vi "Int bottom stacking.vi"() -> (10 "Done":bool)   [LabVIEW 2014]
uses:
  Int Bottom Stacking.ctl
  Bottom Stacking.ctl
panel:
  in  "Int Bottom Stacking":T1
  out "Timer":dbl
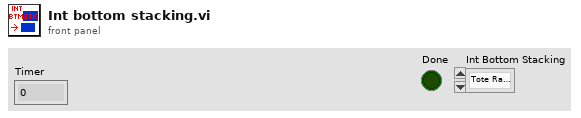
[diagram p1: front panel]
types:
  T1 = typedef "Int Bottom Stacking.ctl" = enum16{"Tote Raising", "Obtaining", "Un-Obtaining", "Tote Lowering", "Tote Release"}
  T2 = typedef "Bottom Stacking.ctl" = enum16{"Tote Raising", "Ejecting", "Un-Ejecting", "Tote Lowering", "Tote Release", "Backing Up"}
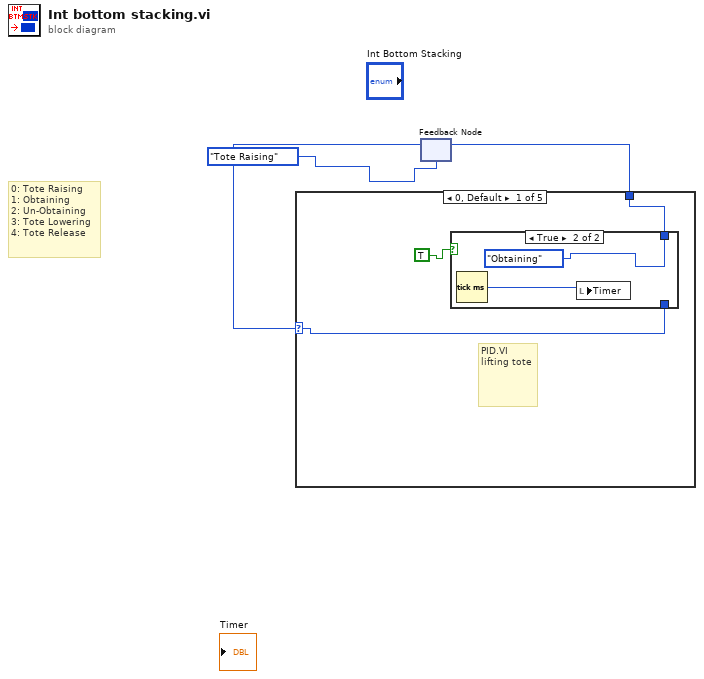
[diagram p0: block diagram]
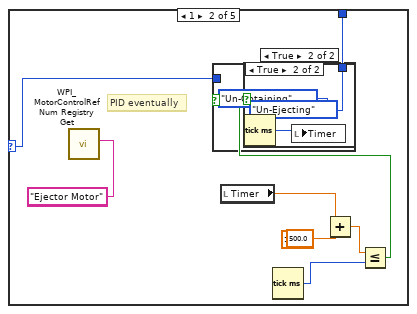
[diagram p3: hidden frame]
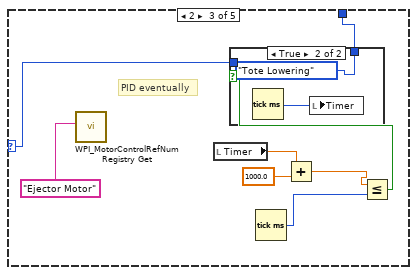
[diagram p6: hidden frame]
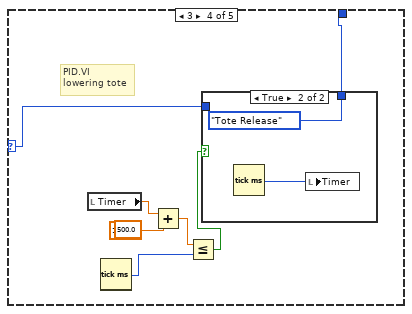
[diagram p8: hidden frame]
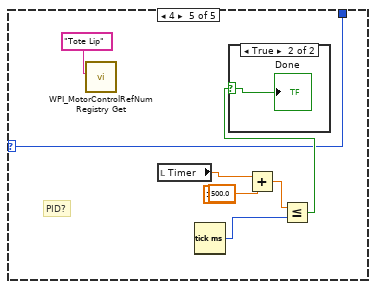
[diagram p10: hidden frame]
diagram:
  # "0: Tote Raising\n1: Obtaining\n2: Un-Obtaining\n3: Tote Lowering\n4: Tote Release"
  n1 = feedback #1(Int_Bottom_Stacking."Tote Raising" ("Int Bottom Stacking")) -> (w3:u16)
  n2 = case shown="0, Default" w3 {
    selector: w3 -> [w5 w10 w27 w37 w47]
    tunnel: [w6 w11 w29 w43 w47] -> w2
    frame 0, Default {
      # "PID.VI\nlifting tote"
      n3 = case shown="True" TRUE {
        tunnel: [w7 Int_Bottom_Stacking."Obtaining" ("Int Bottom Stacking")] -> w6
        tunnel: w5 -> [w7 _]
        frame False {
        }
        frame True {
          n4 = Tick Count (ms)() -> (millisecond timer value=w9:u32)
          n5 = local write "Timer"(w9) -> ()
        }
      }
    }
    frame 1 {
      (unwired) "Ejector Motor" ("refnum name")
      # "PID eventually"
      # "PID eventually"
      n6 = call <vilib>:"WPI_MotorControlRefNum Registry Get.vi"("refnum name"="Ejector Motor") -> ()  [unwired: 9 in, 2 out]
      n7 = local read "Timer"() -> (w21:dbl)
      n8 = local read "Timer"() -> (w12:dbl)
      n9 = Tick Count (ms)() -> (millisecond timer value=w18:u32)
      n10 = Tick Count (ms)() -> (millisecond timer value=w15:u32)
      n11 = Add(x=w21, y=500.0) -> (x+y=w19:dbl)
      n12 = Add(x=w12, y=1000.0) -> (x+y=w14:dbl)
      n13 = Less Or Equal?(x=w19, y=w18) -> (x <= y?=w17:bool)
      n14 = case shown="True" w17 {
        frame False {
        }
        frame True {
          (unwired) Bottom_Stacking."Un-Ejecting" ("Bottom Stacking")
        }
      }
      n15 = Less Or Equal?(x=w14, y=w15) -> (x <= y?=w16:bool)
      n16 = case shown="True" w16 {
        tunnel: [w23 Int_Bottom_Stacking."Un-Obtaining" ("Int Bottom Stacking")] -> w11
        tunnel: w10 -> [w23 _]
        frame False {
        }
        frame True {
          n17 = Tick Count (ms)() -> (millisecond timer value=w25:u32)
          n18 = local write "Timer"(w25) -> ()
        }
      }
    }
    frame 2 {
      # "PID eventually"
      n19 = call <vilib>:"WPI_MotorControlRefNum Registry Get.vi"("refnum name"="Ejector Motor") -> ()  [unwired: 9 in, 2 out]
      n20 = local read "Timer"() -> (w33:dbl)
      n21 = Tick Count (ms)() -> (millisecond timer value=w30:u32)
      n22 = Add(x=w33, y=1000.0) -> (x+y=w31:dbl)
      n23 = Less Or Equal?(x=w31, y=w30) -> (x <= y?=w28:bool)
      n24 = case shown="True" w28 {
        tunnel: [w34 Int_Bottom_Stacking."Tote Lowering" ("Int Bottom Stacking")] -> w29
        tunnel: w27 -> [w34 _]
        frame False {
        }
        frame True {
          n25 = Tick Count (ms)() -> (millisecond timer value=w36:u32)
          n26 = local write "Timer"(w36) -> ()
        }
      }
    }
    frame 3 {
      (unwired) 500.0 ("y")
      # "PID.VI\nlowering tote"
      n27 = local read "Timer"() -> (w39:dbl)
      n28 = Tick Count (ms)() -> ()  [unwired: 1 out]
      n29 = Tick Count (ms)() -> (millisecond timer value=w40:u32)
      n30 = Add(x=w39, y=1000.0) -> (x+y=w41:dbl)
      n31 = Less Or Equal?(x=w41, y=w40) -> (x <= y?=w38:bool)
      n32 = case shown="True" w38 {
        tunnel: [w44 Int_Bottom_Stacking."Tote Release" ("Int Bottom Stacking")] -> w43
        tunnel: w37 -> [w44 _]
        frame False {
        }
        frame True {
          n33 = Tick Count (ms)() -> (millisecond timer value=w46:u32)
          n34 = local write "Timer"(w46) -> ()
        }
      }
    }
    frame 4 {
      (unwired) 1000.0 ("y")
      # "PID?"
      n35 = call <vilib>:"WPI_MotorControlRefNum Registry Get.vi"("refnum name"="Tote Lip") -> ()  [unwired: 9 in, 2 out]
      n36 = local read "Timer"() -> (w49:dbl)
      n37 = Tick Count (ms)() -> (millisecond timer value=w52:u32)
      n38 = Tick Count (ms)() -> ()  [unwired: 1 out]
      n39 = Add(x=w49, y=500.0) -> (x+y=w51:dbl)
      n40 = Less Or Equal?(x=w51, y=w52) -> (x <= y?=w48:bool)
      n41 = case shown="True" w48 {
        selector: w48 -> [_ w54]
        frame False {
        }
        frame True {
          "Done" <- w54
        }
      }
    }
  }
  n42 = feedback-in #1(w2) -> ()
